vi "Calculate Overall Sensor Coverage.vi"(1 "Sensors":map{T1, T2}(c390)) -> (0 "Overall Sensor Coverage":T4(array[cluster]))   [LabVIEW 2020, in "AoC 2022.lvlib"]
uses:
  AoC 2022.lvlib
  <vilib>/4SmartMachines/Polygon Clipping/polyClipping.lvlib
  Location.ctl
  Coverage Area.ctl
  Sensor Info.ctl
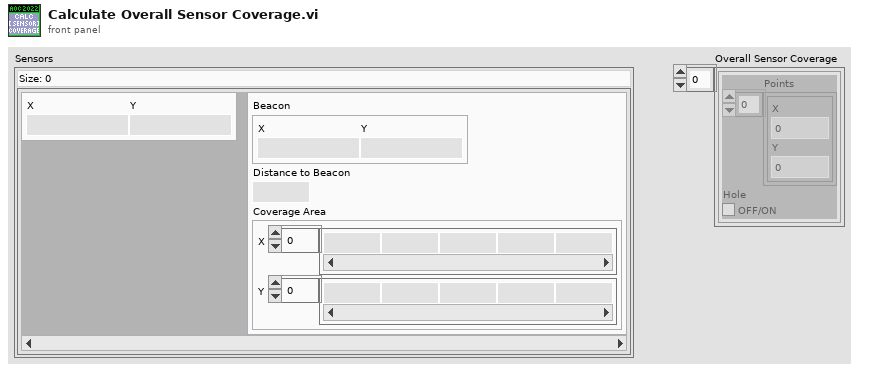
[diagram p1: front panel]
types:
  T1 = typedef "AoC 2022.lvlib/Location.ctl" = cluster{"X":i64, "Y":i64}
  T2 = typedef "AoC 2022.lvlib/Sensor Info.ctl" = cluster{"Beacon":T1, "Distance to Beacon":dbl, "Coverage Area":T3}
  T3 = typedef "AoC 2022.lvlib/Coverage Area.ctl" = cluster{"X":dbl[], "Y":dbl[]}
  T4 = cluster{"Points":cluster{"X":dbl, "Y":dbl}[], "Hole":bool}[]
  T5 = enum16{"Intersection", "Union", "Difference", "Xor"}
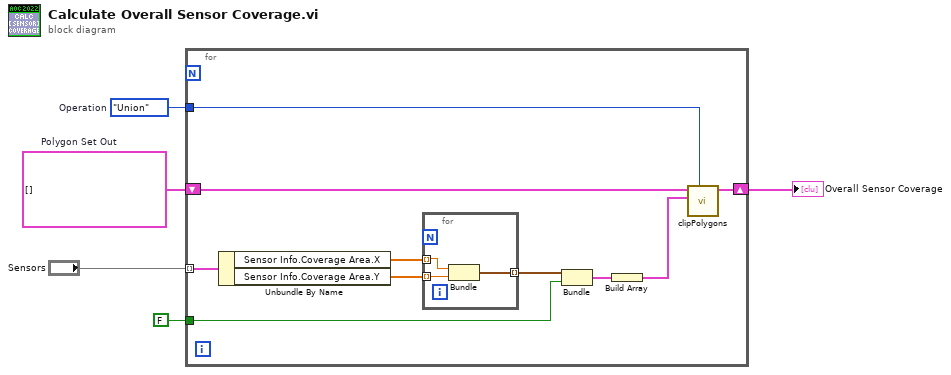
[diagram p0: block diagram]
diagram:
  w4 = T5."Union"  # Operation
  w2 = T4 []  # Polygon Set Out
  n1 = for {
    tunnel: "Sensors" -> [w15] mode=indexing
    shift-right: [w14] -> w5
    shift-left: w2 -> [w13]
    tunnel: FALSE -> [w12]
    tunnel: w4 -> [w9]
    n2 = Unbundle By Name(w15) -> ("Sensor Info.Coverage Area.X"=w7:dbl[], "Sensor Info.Coverage Area.Y"=w6:dbl[])
    n3 = for {
      tunnel: w7 -> [w18] mode=indexing
      tunnel: w6 -> [w17] mode=indexing
      tunnel: [w16] -> w8 mode=indexing
      n4 = Bundle("X"=w18, "Y"=w17) -> (w16:cluster{"X":dbl, "Y":dbl})  [unwired: 1 in]
    }
    n5 = Bundle(w8, w12) -> (w11:cluster{cluster{"X":dbl, "Y":dbl}[], bool})  [unwired: 1 in]
    n6 = Build Array(w11) -> (w10:cluster{cluster{"X":dbl, "Y":dbl}[], bool}[])
    n7 = call <vilib>:"clipPolygons.vi"("Operation"=w9, "Polygon Set 2"=w10, "Polygon Set 1"=w13) -> ("Polygon Set Out"=w14:T4)  [unwired: 7 in, 1 out]
  }
  "Overall Sensor Coverage" <- w5
